vi "Reset Counts.vi"(8 "error in (no error)":errorcluster, 11 "TrafficMap in":refnum<class "TrafficMap.lvclass">) -> (0 "error out":errorcluster, 3 "TrafficMap out":refnum<class "TrafficMap.lvclass">)   [LabVIEW 2017, in "TrafficMap.lvclass"]
uses:
  TrafficMap.lvclass
  TrafficMap.lvclass/TrafficMap.ctl
  Zone/Zone.lvclass/Zone.ctl
  Zone/Zone.lvclass
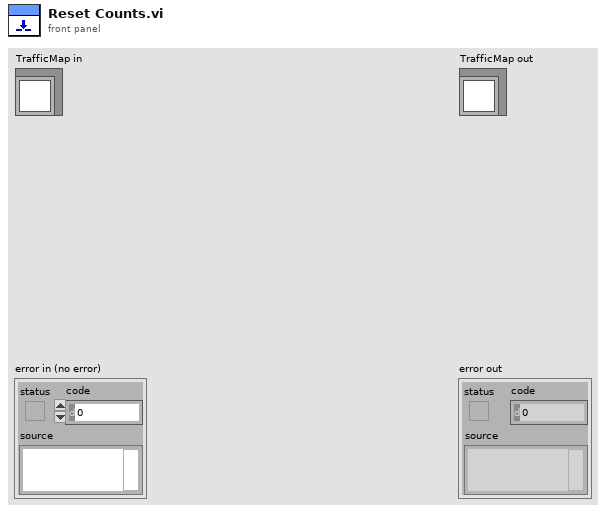
[diagram p1: front panel]
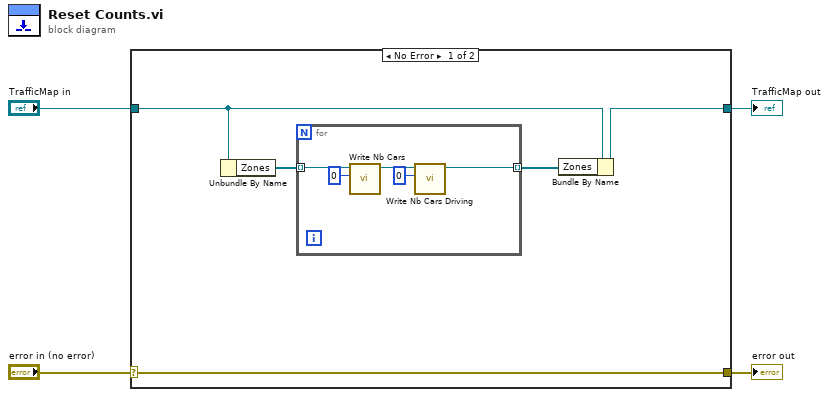
[diagram p0: block diagram]
diagram:
  n1 = case shown="No Error" "error in (no error)" {
    selector: "error in (no error)" -> [w9 w16]
    tunnel: [w9 w16] -> w3
    tunnel: [w7 w15] -> w1
    tunnel: "TrafficMap in" -> [w8 w15]
    frame No Error {
      n2 = Unbundle By Name(w8) -> ("Zones"=w6:refnum<class "Zone.lvclass">[])
      n3 = for {
        tunnel: w6 -> [w14] mode=indexing
        tunnel: [w12] -> w5 mode=indexing
        n4 = call "Write Nb Cars.vi"("Nb Cars"=u32 0, "Zone in"=w14) -> ("Zone out"=w13:refnum<class "Zone.lvclass">)  [unwired: 8 in, 1 out]
        n5 = call "Write Nb Cars Driving.vi"("Nb Cars Driving"=u32 0, "Zone in"=w13) -> ("Zone out"=w12:refnum<class "Zone.lvclass">)  [unwired: 8 in, 1 out]
      }
      n6 = Bundle By Name(cluster=w8, "Zones"=w5) -> (w7:refnum<class "TrafficMap.lvclass">)
    }
    frame Error {
    }
  }
  "error out" <- w3
  "TrafficMap out" <- w1
